vi "Log Plot Save-Recall Setup.vi"(6 "Memory Location":path, 8 "error in (no error)":errorcluster, 9 "Trace (1:Trace 1)":u16(ring)=1 items=["Trace 1"=1, "Trace 2"=2, "Trace 3"=3], 10 "Operation (0: Load Log Plot Trace)":u16(ring) items=["Load Log Plot Trace", "Save Log Plot Trace"], 11 "VISA resource name":refnum<visa-resource-name>) -> (0 "error out":errorcluster, 3 "VISA resource name out":refnum<visa-resource-name>)   [LabVIEW 2014, in "Agilent ESA PSA Series.lvlib"]
doc: "Saves or restores reference traces to or from the device storage.\n\n<B>Note:</B>\n\nThis VI is only valid in Phase Noise personality. Use <B>Switch Personality</B> VI to switch to Phase Noise before calling this VI."
uses:
  Agilent ESA PSA Series.lvlib
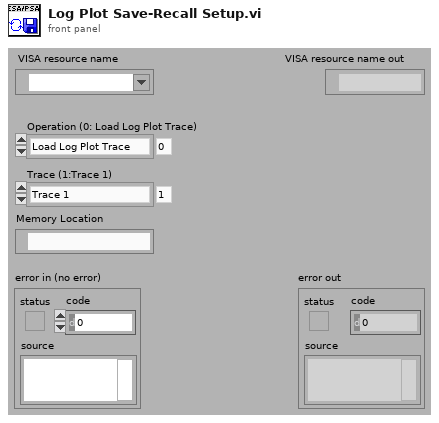
[diagram p1: front panel]
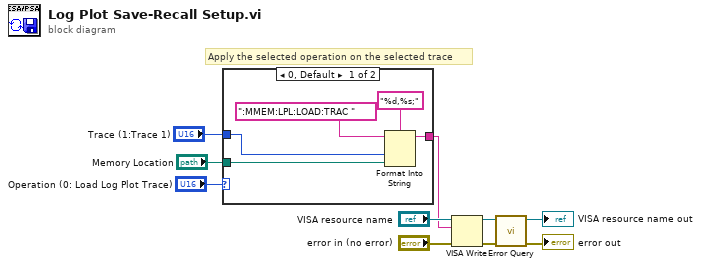
[diagram p0: block diagram]
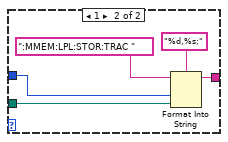
[diagram p2: hidden frame]
diagram:
  # "Apply the selected operation on the selected trace"
  n1 = case shown="0, Default" "Operation (0: Load Log Plot Trace)" {
    tunnel: "Memory Location" -> [w13 w19]
    tunnel: "Trace (1:Trace 1)" -> [w12 w20]
    tunnel: [w11 w18] -> w1
    frame 0, Default {
      n2 = Format Into String(format string="%d,%s;", initial string=":MMEM:LPL:LOAD:TRAC ", w12, w13) -> (resulting string=w11:string)  [unwired: 1 in, 1 out]
    }
    frame 1 {
      n3 = Format Into String(format string="%d,%s;", initial string=":MMEM:LPL:STOR:TRAC ", w20, w19) -> (resulting string=w18:string)  [unwired: 1 in, 1 out]
    }
  }
  n4 = VISA Write(VISA resource name="VISA resource name", write buffer=w1, error in (no error)="error in (no error)") -> (VISA resource name out=w3:refnum<visa-resource-name>, error out=w2:errorcluster)  [unwired: 1 out]
  n5 = call "Error Query.vi"("error in (no error)"=w2, "VISA resource name"=w3) -> ("error out"=→"error out":errorcluster, "VISA resource name out"=→"VISA resource name out":refnum<visa-resource-name>)  [unwired: 6 in, 2 out]
